vi "ADC Get Data.vi"(9 "BufferSize":i32, 10 "pDataBuffer":u16, 11 "DevIndex":i32) -> (2 "pDataBuffer out":u16, 3 "function return":i32)   [LabVIEW 2010, in "usb2adc.lvlib"]
doc: "int WINAPI ADC_GetData(int DevIndex,unsigned short *pDataBuffer,int BufferSize);"
uses:
  usb2adc.lvlib
  USB2XXX.dll
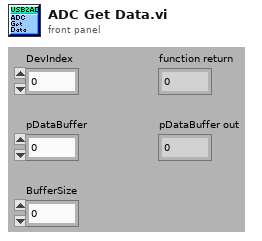
[diagram p1: front panel]
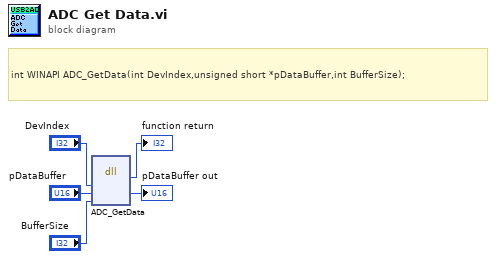
[diagram p0: block diagram]
diagram:
  # "int WINAPI ADC_GetData(int DevIndex,unsigned short *pDataBuffer,int BufferSize);"
  n1 = dll-call lib="G:/OtherWork/USB2XXX_Example/trunk/Labview/PublicFiles/usb2adc/USB2XXX.*" fn="ADC_GetData"("DevIndex"="DevIndex", "pDataBuffer"="pDataBuffer", "BufferSize"="BufferSize") -> (→"function return":i32, "pDataBuffer"=→"pDataBuffer out":u16)  [unwired: 5 in, 2 out]
